vi "LINX_read_temp.vi"(6 "n_step":refnum<vi>, 7 "n_avg":i32=1000, 8 "Error In":errorcluster, 11 "LINX Resource":T1={"IO"=enum."Remote", "Interface"=enum."Serial", "LINX Device Config"={"Interface"=enum."Serial", "COM Port"="COM25", "TCP Configuration"={"IP Address"="", "Port"=0}, "Device Family"=2, "Device ID"=0, "Device Name"="Arduino Uno\u0000", "TCP Ref"=refnum, "Channels"={"DI"=[0, 1, 2, 3, 4, 5, 6, 7, 8, 9, 10, 11, 12, 13, 14, 15, 16, 17, 18, 19], "DO"=[0, 1, 2, 3, 4, 5, 6, 7, 8, 9, 10, 11, 12, 13, 14, 15, 16, 17, 18, 19], "AI"=[0, 1, 2, 3, 4, 5], "AO"=[], "PWM"=[3, 5, 6, 9, 10, 11], "QE"=[], "UART"=[0], "I2C 2"=[0], "SPI"=[0], "CAN"=[], "Servo"=[0, 1, 2, 3, 4, 5, 6, 7, 8, 9, 10, 11, 12, 13, 14, 15, 16, 17, 18, 19], "AI Ref (V)"=5.0, "AI Resolution (Bits)"=0, "AO Ref (V)"=0.0, "AO Resolution (Bits)"=0}}}) -> (0 "Error Out":errorcluster, 1 "status":bool=TRUE, 2 "array_flow":dbl[](array[numeric]), 3 "LINX Resource Out":T1={"IO"=enum."Remote", "Interface"=enum."Serial", "LINX Device Config"={"Interface"=enum."Serial", "COM Port"="COM25", "TCP Configuration"={"IP Address"="", "Port"=0}, "Device Family"=2, "Device ID"=0, "Device Name"="Arduino Uno\u0000", "TCP Ref"=refnum, "Channels"={"DI"=[0, 1, 2, 3, 4, 5, 6, 7, 8, 9, 10, 11, 12, 13, 14, 15, 16, 17, 18, 19], "DO"=[0, 1, 2, 3, 4, 5, 6, 7, 8, 9, 10, 11, 12, 13, 14, 15, 16, 17, 18, 19], "AI"=[0, 1, 2, 3, 4, 5], "AO"=[], "PWM"=[3, 5, 6, 9, 10, 11], "QE"=[], "UART"=[0], "I2C 2"=[0], "SPI"=[0], "CAN"=[], "Servo"=[0, 1, 2, 3, 4, 5, 6, 7, 8, 9, 10, 11, 12, 13, 14, 15, 16, 17, 18, 19], "AI Ref (V)"=5.0, "AI Resolution (Bits)"=0, "AO Ref (V)"=0.0, "AO Resolution (Bits)"=0}}}, 4 "array_voltage":dbl[](array[numeric]))   [LabVIEW 2019]
uses:
  <vilib>/MakerHub/LINX/Private/Type Defs/LINX Ref.ctl
  <vilib>/MakerHub/LINX/Private/Type Defs/Platform.ctl
  <vilib>/MakerHub/LINX/Private/Type Defs/Interface.ctl
  <vilib>/MakerHub/LINX/Private/Device/Type Defs/LINX Device Config.ctl
  <vilib>/MakerHub/LINX/Private/Device/Type Defs/TCP Config.ctl
  <vilib>/MakerHub/LINX/Private/Device/Type Defs/Channels.ctl
  <vilib>/MakerHub/LINX/Public/Peripherals/Analog/Analog Read N Chans.vi
  <vilib>/Analysis/baseanly.llb/Mean (DBL).vi
  <vilib>/MakerHub/LINX/Private/Local IO/LinxAnalogRead.vi
  <vilib>/MakerHub/LINX/Public/Utilities/Check Channel.vi
  <vilib>/MakerHub/LINX/Private/Utilties/Generate Error.vi
  <vilib>/MakerHub/LINX/LMH-LINX.lvlib
  <vilib>/Analysis/NI_AALBase.lvlib
  <vilib>/MakerHub/LINX/Private/Device/Device.lvlib
panel:
  in  "conv_p1":dbl[](array[numeric])=[1.42, 1.42, 1.42, 1.42, 1.42]
  in  "conv_p0":dbl[](array[numeric])=[0.3, 0.3, 0.3, 0.3, 0.3]
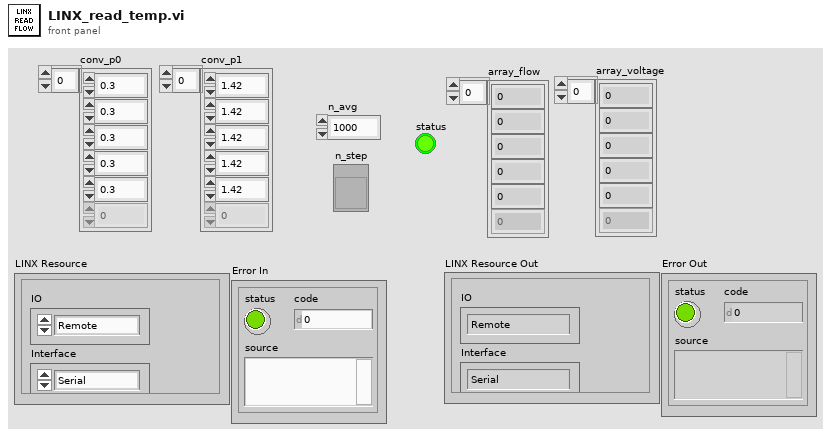
[diagram p1: front panel]
types:
  T1 = typedef "LMH-LINX.lvlib/LINX Ref.ctl" = cluster{"IO":T2, "Interface":T3, "LINX Device Config":T4}
  T2 = typedef "LMH-LINX.lvlib/Platform.ctl" = enum16{"Remote", "Local"}
  T3 = typedef "LMH-LINX.lvlib/Interface.ctl" = enum16{"Serial", "TCP"}
  T4 = typedef "LMH-LINX.lvlib/Device.lvlib/LINX Device Config.ctl" = cluster{"Interface":T3, "COM Port":refnum<visa-resource-name>, "TCP Configuration":T5, "Device Family":u8, "Device ID":u8, "Device Name":string, "TCP Ref":refnum<k5>, "Channels":T6}
  T5 = typedef "LMH-LINX.lvlib/Device.lvlib/TCP Config.ctl" = cluster{"IP Address":string, "Port":u16}
  T6 = typedef "LMH-LINX.lvlib/Channels.ctl" = cluster{"DI":u8[], "DO":u8[], "AI":u8[], "AO":u8[], "PWM":u8[], "QE":u8[], "UART":u8[], "I2C 2":u8[], "SPI":u8[], "CAN":u8[], "Servo":u8[], "AI Ref (V)":dbl, "AI Resolution (Bits)":u8, "AO Ref (V)":dbl, "AO Resolution (Bits)":u8}
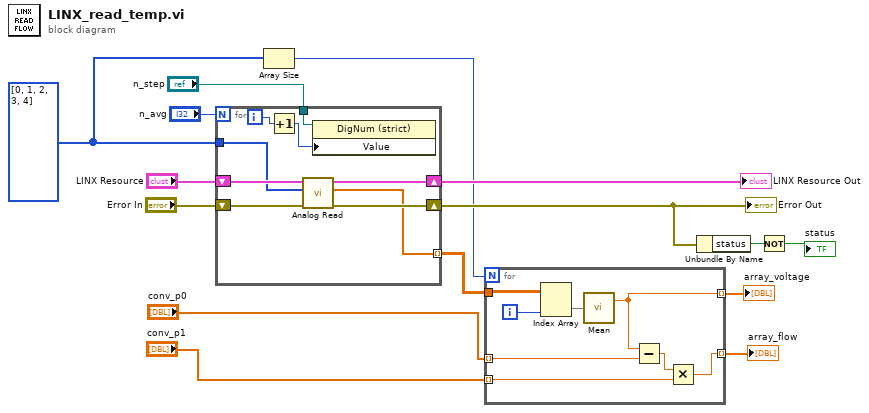
[diagram p0: block diagram]
diagram:
  w1 = u8[] [0, 1, 2, 3, 4] ("AI Channel(s)")
  n1 = for {
    N: "n_avg" -> [_]
    tunnel: [w20] -> w8 mode=indexing
    shift-right: [w22] -> w13
    shift-left: "LINX Resource" -> [w24]
    shift-right: [w21] -> w12
    shift-left: "Error In" -> [w23]
    tunnel: "n_step" -> [w19]
    tunnel: w1 -> [w16]
    i -> [w18]
    n2 = Increment(x=w18) -> (x+1=w17:i32)
    n3 = call-poly <vilib>:"Analog Read.vi"("Error In"=w23, "AI Channel(s)"=w16, "LINX Resource"=w24) -> ("Error Out"=w21:errorcluster, "Voltages"=w20:dbl[], "LINX Resource"=w22:T1)  [unwired: 5 in, 1 out]
    n4 = property class="DigNum (strict)"(reference=w19, "Value"=w17) -> ()  [unwired: 1 in, 2 out]
  }
  "LINX Resource Out" <- w13
  "Error Out" <- w12
  n5 = Array Size(array=w1) -> (size(s)=w6:i32)
  n6 = for {
    N: w6 -> [_]
    tunnel: w8 -> [w32]
    tunnel: [w26] -> w7 mode=indexing
    tunnel: [w29] -> w5 mode=indexing
    tunnel: "conv_p0" -> [w28] mode=indexing
    tunnel: "conv_p1" -> [w27] mode=indexing
    i -> [w31]
    n7 = Index Array(array=w32, index (col)=w31) -> (element=w30:dbl[])  [unwired: 1 in]
    n8 = call-poly <vilib>:"Mean.vi"("X"=w30) -> ("mean"=w29:dbl)  [unwired: 1 out]
    n9 = Subtract(x=w29, y=w28) -> (x-y=w25:dbl)
    n10 = Multiply(x=w25, y=w27) -> (x*y=w26:dbl)
  }
  "array_flow" <- w7
  "array_voltage" <- w5
  n11 = Unbundle By Name(w12) -> ("status"=w11:bool)
  n12 = Not(x=w11) -> (.not. x?=→"status":bool)
